vi "G4BaseTemplate_Singleton_6x8x6_ReadWriteAttribute.vi"(5 "Error In":errorcluster) -> (19 "Error Out":errorcluster)   [LabVIEW 2020]
uses:
  <resource>/Framework/Providers/Open_GDS/ClassProviders/Provider_EndevoGOOP400/Templates/G4BaseTemplate_Singleton_6x8x6/G4BaseTemplate_Singleton_6x8x6.lvclass
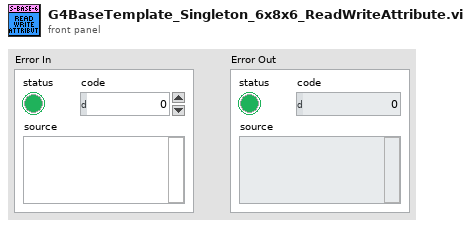
[diagram p1: front panel]
types:
  T1 = typedef "G4BaseTemplate_Singleton_6x8x6.lvclass/ObjectAttributes.ctl" = cluster{"Attribute1":dbl}
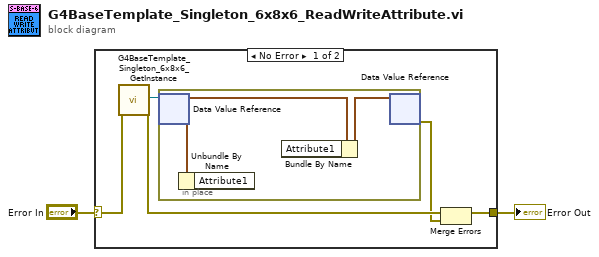
[diagram p0: block diagram]
diagram:
  n1 = case shown="No Error" "Error In" {
    selector: "Error In" -> [w6 w10]
    tunnel: [w7 w10] -> w1
    frame No Error {
      n2 = call <resource>:"G4BaseTemplate_Singleton_6x8x6_GetInstance.vi"("Error In"=w6) -> ("DVRRefOut"=w5:refnum<data-value>, "Error Out"=w4:errorcluster)  [unwired: 14 in, 3 out]
      n3 = in-place {
        n4 = in-place-dvr #1(w5) -> (w8:T1)  [unwired: 1 out]
        n5 = Unbundle By Name(w8) -> ()  [unwired: 1 out]
        n6 = Bundle By Name(cluster=w8) -> (w9:T1)  [unwired: 1 in]
        n7 = in-place-dvr #1(w9) -> (w3:errorcluster)  [unwired: 1 out]
      }
      n8 = Merge Errors(w4, w3) -> (w7:errorcluster)
    }
    frame Error {
    }
  }
  "Error Out" <- w1
